vi "DeepLabv3_OpenVINO.vi"() -> ()   [LabVIEW 2018]
doc: "DeepLabv3_OpenVINO: This example is a semantic segmentation example of the DeepLabv3 model, which can be used for image semantic segmentation tasks. The ability to segment videos into semantically meaningful regions and assign a semantic label to each pixel."
uses:
  vi.lib/VIRobotics/ModelZoo/Segmentation/Yiku_Seg_OpenVINO/InitialModel_deeplabv3_OpenVINO.vi
  vi.lib/VIRobotics/ModelZoo/Segmentation/Yiku_Seg_OpenVINO/Yiku_Seg_OpenVINO.lvclass
  vi.lib/VIRobotics/opencv_yiku/Cap/Cap.lvclass
panel:
  in  "class_names_path":path=path "C:/ProgramData/VIRobotics/ModelZoo/Segmentation/class.txt"
  in  "device_name":string(combo)="CPU"
  in  "model_file":path
  in  "stop":bool
  out "picture":picture
  out "每帧耗时(s)":dbl
  out "mask":picture
  # "Overview: Demonstrates how to use OpenVINO to load the ONNX model of deeplabv3 for real-time image segmentation.\nRequirements: Windows.\nMake sure your computer has a camera。\nInstructions: \nInstructions: \n1.Select the device_name to use.（If your computer has Intel GPU, you can select GPU in the \"type\" control before running the VI to achieve faster inference).\n2.Download the model of deeplabv3.Specify the model_file ,then run the VI.\nIf you want to load the model you trained, follow the following steps:\n1.Select the device_name to use. \n2.Specify the model_file and class_names_file.\n3.Run the VI."
  # "Download the model of deeplabv3"
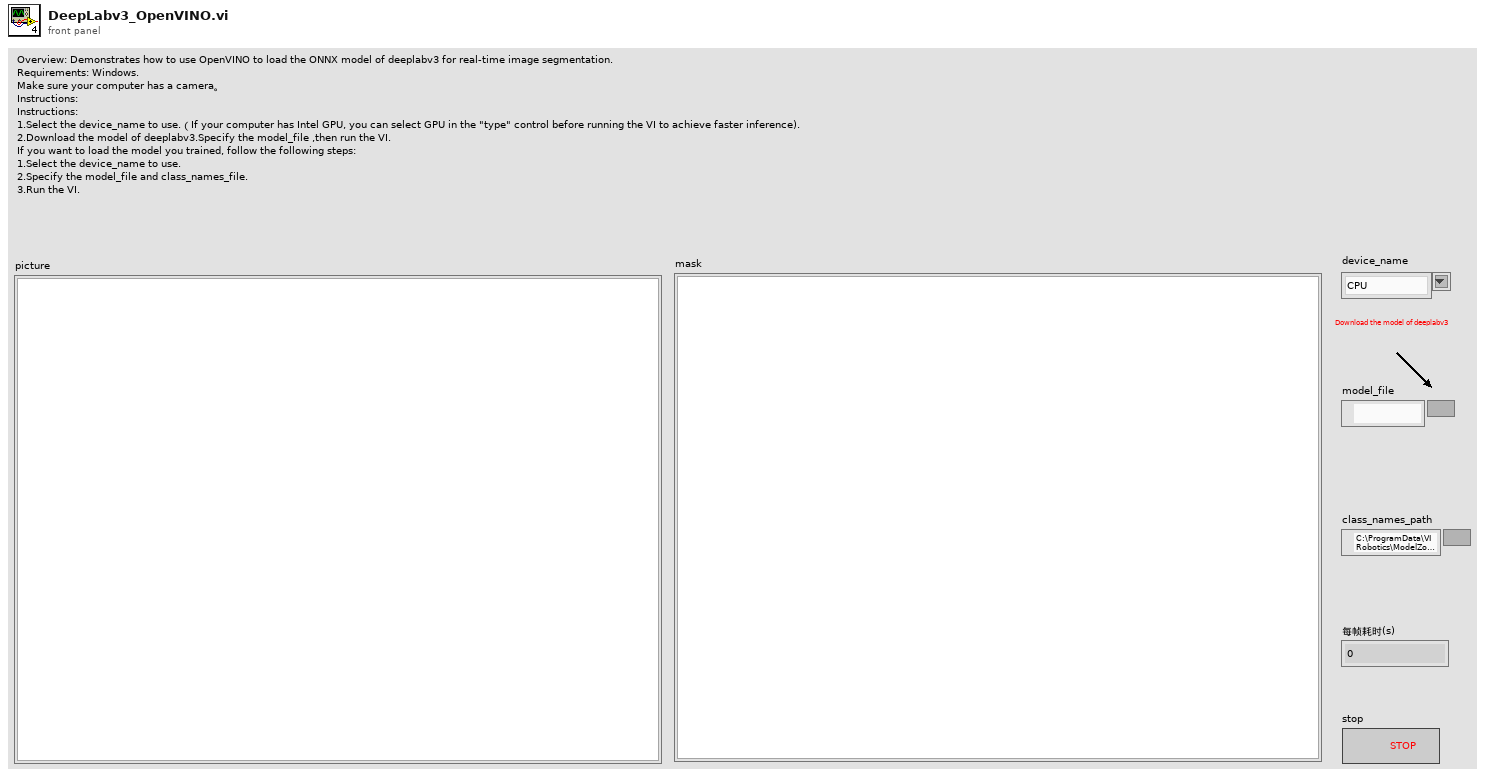
[diagram p1: front panel]
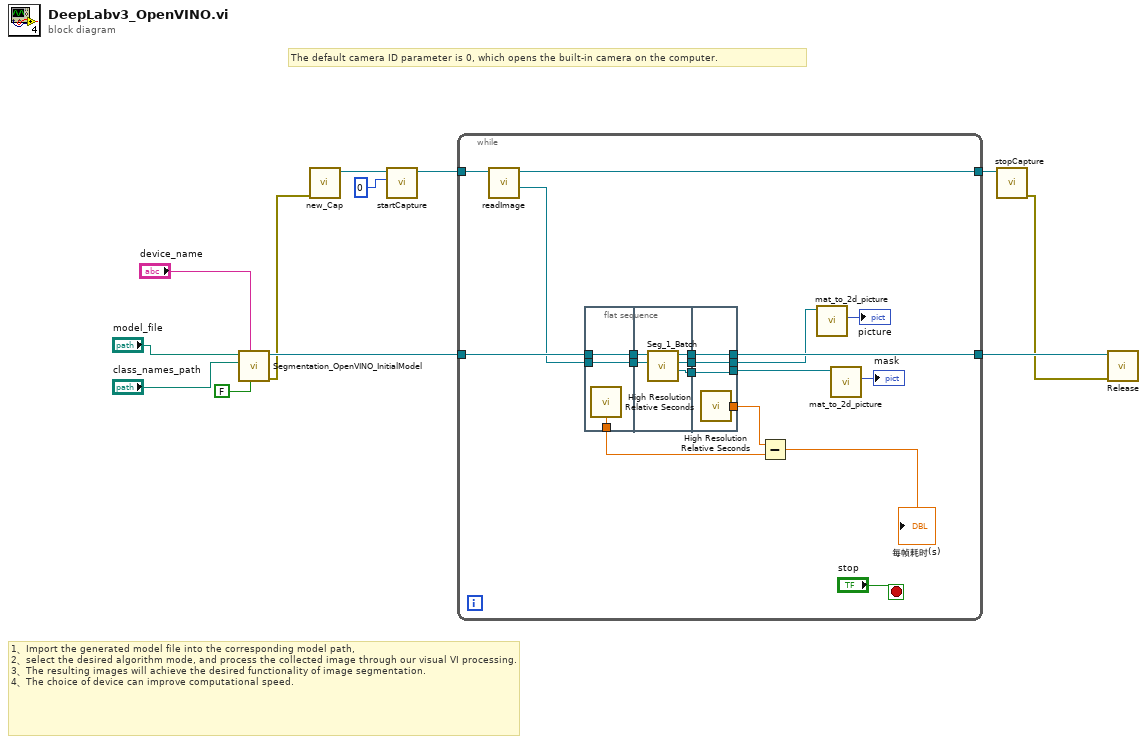
[diagram p0: block diagram]
diagram:
  # "1、Import the generated model file into the corresponding model path, \n2、select the desired algorithm mode, and process the collected image through our visual VI processing. \n3、The resulting images will achieve the desired functionality of image segmentation. \n4、The choice of device can improve computational speed."
  # "The default camera ID parameter is 0, which opens the built-in camera on the computer."
  n1 = call-poly "Segmentation_OpenVINO_InitialModel.vi"("use letterbox"=FALSE, "device_name"="device_name", "class_names_path"="class_names_path", "path"="model_file") -> ("error out"=w6:errorcluster, "Seg_OV out"=w7:refnum<class "Yiku_Seg_OpenVINO.lvclass">)  [unwired: 6 in]
  n2 = call "new_Cap.vi"("error in (no error)"=w6) -> ("Cap out"=w12:refnum<class "Cap.lvclass">)  [unwired: 9 in, 1 out]
  n3 = call "startCapture.vi"("cameraID"=0, "Cap in"=w12) -> ("Cap out"=w11:refnum<class "Cap.lvclass">)  [unwired: 8 in, 1 out]
  n4 = while {
    tunnel: w11 -> [w30]
    tunnel: [w29] -> w10
    tunnel: w7 -> [w27]
    tunnel: [w25] -> w9
    stop <- "stop" stop-if-true
    n5 = call "readImage.vi"("Cap in"=w30) -> ("Mat out"=w26:refnum<class "Mat_8U.lvclass">, "Cap out"=w29:refnum<class "Cap.lvclass">)  [unwired: 8 in, 1 out]
    n6 = flat-sequence {
      tunnel: w26 -> [w32]
      tunnel: w27 -> [w33]
      tunnel: [w33] -> w22
      tunnel: [w32] -> w21
      tunnel: [w31] -> w17
      tunnel: w22 -> [w38]
      tunnel: w21 -> [w37]
      tunnel: [w36] -> w20
      tunnel: [w35] -> w19
      tunnel: [w34] -> w14
      tunnel: [w41] -> w24
      tunnel: [w42] -> w25
      tunnel: w20 -> [w42]
      tunnel: w19 -> [w41]
      tunnel: [w40] -> w18
      tunnel: [w39] -> w13
      tunnel: w14 -> [w39]
      frame #0 {
        n7 = call <vilib>:"High Resolution Relative Seconds.vi"() -> ("relative seconds"=w31:dbl)
      }
      frame #1 {
        n8 = call-dynamic "Seg_1_Batch.vi"("img"=w37, "Seg_OV in"=w38) -> ("mask"=w34:refnum<class "Mat_8U.lvclass">, "img out"=w35:refnum<class "Mat_8U.lvclass">, "Seg_OV out"=w36:refnum<class "Yiku_Seg_OpenVINO.lvclass">)  [unwired: 6 in, 1 out]
      }
      frame #2 {
        n9 = call <vilib>:"High Resolution Relative Seconds.vi"() -> ("relative seconds"=w40:dbl)
      }
    }
    n10 = Subtract(x=w18, y=w17) -> (x-y=→"每帧耗时(s)":dbl)
    n11 = call "mat_to_2d_picture.vi"("Mat_8U in"=w24) -> ("picture"=→"picture":picture)  [unwired: 8 in, 2 out]
    n12 = call "mat_to_2d_picture.vi"("Mat_8U in"=w13) -> ("picture"=→"mask":picture)  [unwired: 8 in, 2 out]
  }
  n13 = call "stopCapture.vi"("Cap in"=w10) -> ("error out"=w8:errorcluster)  [unwired: 10 in]
  n14 = call-dynamic "Release.vi"("error in (no error)"=w8, "Seg_OV in"=w9) -> ()  [unwired: 8 in, 2 out]
